vi "image二值化（子VI）.vi"(1 "阈值设置":u8, 2 "Image Dst":T1, 3 "Image Src":T1) -> (0 "Image Out":T1)   [LabVIEW 2017]
uses:
  <vilib>/vision/Image Controls.llb/IMAQ Image.ctl
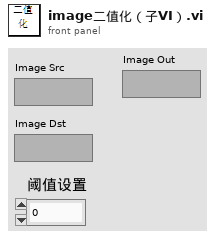
[diagram p1: front panel]
types:
  T1 = typedef "IMAQ Image.ctl" = refnum<image>
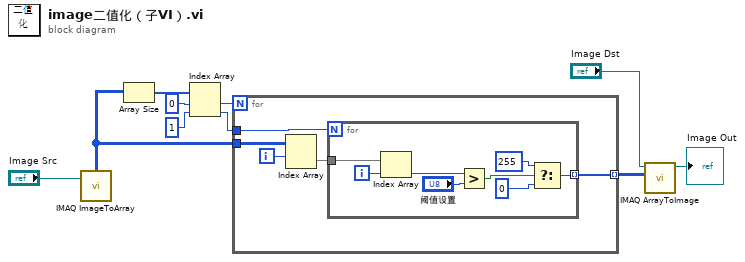
[diagram p0: block diagram]
diagram:
  n1 = call "IMAQ ImageToArray"("Image"="Image Src") -> ("Image Pixels (U8)"=w7:u8[][])  [unwired: 2 in, 5 out]
  n2 = Array Size(array=w7) -> (size(s)=w6:i32[])
  n3 = Index Array(array=w6, index #1=0 ("索引"), index #2=1 ("索引")) -> (element #1=w5:i32, element #2=w1:i32)
  n4 = for {
    N: w5 -> [_]
    tunnel: w7 -> [w15]
    tunnel: w1 -> [w13]
    tunnel: [w11] -> w10 mode=indexing
    i -> [w14]
    n5 = Index Array(array=w15, index (row)=w14) -> (element=w12:u8[])  [unwired: 1 in]
    n6 = for {
      N: w13 -> [_]
      tunnel: w12 -> [w23]
      tunnel: [w19] -> w11 mode=indexing
      i -> [w22]
      n7 = Index Array(array=w23, index=w22) -> (element=w21:u8)
      n8 = Greater?(x=w21, y="阈值设置") -> (0:w20:bool)
      n9 = Select(t=255, s=w20, f=0) -> (s? t:f=w19:i32)
    }
  }
  n10 = call "IMAQ ArrayToImage"("Image Pixels (U8)"=w10, "Image"="Image Dst") -> ("Image Out"=→"Image Out":T1)  [unwired: 4 in, 5 out]
